vi "mlink_scan_trigger_external_start.vi"(7 "trigger type":T2, 8 "error in (no error)":errorcluster, 10 "source":T1 items=["AO_Start", "AI_Start", "DSP_Start"], 11 "connection ID":i32=-1) -> (0 "error out":errorcluster, 3 "connection ID out":i32)   [LabVIEW 2009, in "MicroDAQ.lvlib" / "mlink.lvlib"]
uses:
  <instrlib>/MicroDAQ/Mlink library wraper/mlink.lvlib
  <instrlib>/MicroDAQ/Tools/Trigger type.ctl
  <instrlib>/MicroDAQ/Tools/External start trigger source.ctl
  <instrlib>/MicroDAQ/MLink32.dll
  <instrlib>/MicroDAQ/MicroDAQ.lvlib
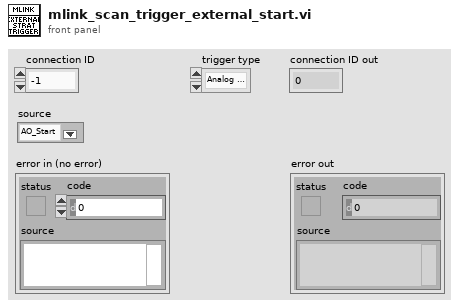
[diagram p1: front panel]
types:
  T1 = typedef "MicroDAQ.lvlib/External start trigger source.ctl" = u8
  T2 = typedef "MicroDAQ.lvlib/Trigger type.ctl" = enum8{"Analog output", "Analog input"}
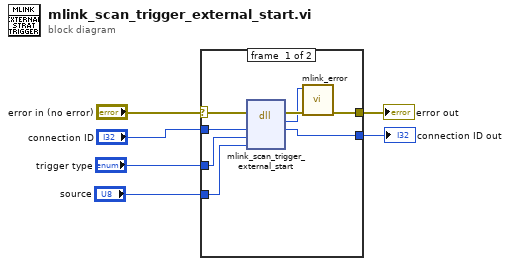
[diagram p0: block diagram]
diagram:
  n1 = case shown="No Error" "error in (no error)" {
    selector: "error in (no error)" -> [w14 w16]
    tunnel: "connection ID" -> [w13 w15]
    tunnel: [w12 w15] -> w4
    tunnel: [w9 w16] -> w3
    tunnel: "trigger type" -> [w8 _]
    tunnel: "source" -> [w7 _]
    frame #0 {
      n2 = dll-call lib="C:/Program Files (x86)/National Instruments/LabVIEW 2009/instr.lib/MicroDAQ/MLink32.dll" fn="mlink_scan_trigger_external_start" ("MLink64.dll:mlink_dsp_run")(error in=w14, "link_fd"=w13, "trigger"=w8, "source"=w7) -> (error out=w11:errorcluster, "return type"=w10:i32, "link_fd"=w12:i32)  [unwired: 4 in, 1 out]
      n3 = call <instrlib>:"mlink_error.vi"("error in (no error)"=w11, "error code"=w10) -> ("error out"=w9:errorcluster)  [unwired: 9 in]
    }
    frame #1 {
    }
  }
  "connection ID out" <- w4
  "error out" <- w3
